vi "Set HW data.vi"(4 "Slot":T1) -> (1 "HW DATA":string)   [LabVIEW 2013]
uses:
  SystemCode/SysControl/Slot.ctl
  CCID info.ctl
  GlobalValue.vi
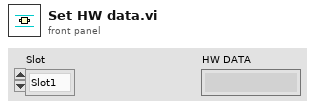
[diagram p1: front panel]
types:
  T1 = typedef "Slot.ctl" = enum16{"Slot1", "Slot2", "Slot3", "Slot4"}
  T2 = typedef "CCID info.ctl" = enum16{"Fw Ver", "HW Ver", "CCID", "WiFiName", "DevID"}
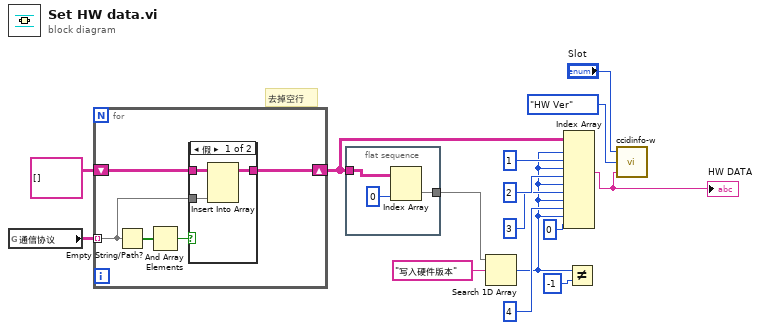
[diagram p0: block diagram]
diagram:
  # "去掉空行"
  n1 = global read "GlobalValue.vi" "通信协议"() -> (w2:string[][])
  n2 = for {
    tunnel: w2 -> [w16] mode=indexing
    shift-right: [w19] -> w8
    shift-left: string[][] [] -> [w20]
    n3 = Empty String/Path?(string/path=w16) -> (empty?=w18:bool[])
    n4 = And Array Elements(Boolean array=w18) -> (logical AND=w17:bool)
    n5 = case shown="假" w17 {
      tunnel: w20 -> [w23 w24]
      tunnel: [w22 w24] -> w19
      tunnel: w16 -> [w21 _]
      frame False {
        n6 = Insert Into Array(array=w23, new element=w21) -> (w22:string[][])  [unwired: 2 in]
      }
      frame True {
      }
    }
  }
  n7 = flat-sequence {
    tunnel: [w26] -> w11
    tunnel: w8 -> [w25]
    frame #0 {
      n8 = Index Array(array=w25, index (col)=0 ("禁用的索引 (列)")) -> (element=w26:string[])  [unwired: 1 in]
    }
  }
  n9 = Search 1D Array(1D array=w11, element="写入硬件版本" ("通信协议名称")) -> (index of element=w7:i32)  [unwired: 1 in]
  n10 = Index Array(array=w8, index (row) #1=w7, index (col) #1=1 ("索引 (列)"), index (row) #2=w7, index (col) #2=2 ("索引 (列)"), index (row) #3=w7, index (col) #3=3 ("索引 (列)"), index (row) #4=w7, index (col) #4=4 ("禁用的索引 (列)"), index (row) #5=w7, index (col) #5=0 ("禁用的索引 (列)")) -> (element #2=w3:string)  [unwired: 4 out]
  "HW DATA" <- w3
  n11 = Not Equal?(x=w7, y=-1) -> ()  [unwired: 1 out]
  n12 = call "ccidinfo-w.vi"("Data"=w3, "Data Type"=CCID_info."HW Ver", "Slot"="Slot") -> ()  [unwired: 1 in]
